vi "Class Data Type.vi"(8 "error in (no error)":errorcluster, 11 "Group in":refnum<class "Group.lvclass">) -> (0 "error out":errorcluster, 2 "Class Data Type":T1, 3 "Group out":refnum<class "Group.lvclass">)   [LabVIEW 2020, in "Vecto.lvlib" / "Group.lvclass"]
uses:
  Group.lvclass
  Group Data Type.ctl
  VectoConfig/VectoConfig.lvlib
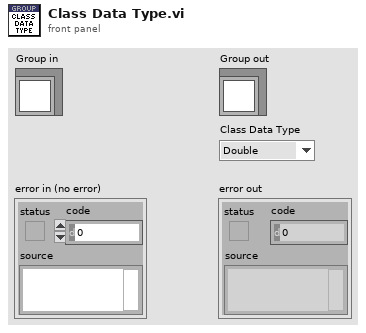
[diagram p1: front panel]
types:
  T1 = typedef "VectoConfig.lvlib/Group Data Type.ctl" = enum16{"Double", "String", "Bool"}
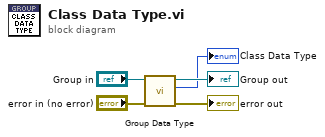
[diagram p0: block diagram]
diagram:
  n1 = call-dynamic "Group Data Type.vi"("error in (no error)"="error in (no error)", "Group in"="Group in") -> ("error out"=→"error out":errorcluster, "Group Data Type"=→"Class Data Type":T1, "Group out"=→"Group out":refnum<class "Group.lvclass">)  [unwired: 7 in]
